vi "GenerateSelectorBounds.vi"(8 "error in (no error)":errorcluster, 10 "Master Bounds Rect":T1, 11 "MultiFrameStructure in":refnum<vi>) -> (0 "error out":errorcluster, 2 "JSON string":string, 3 "reference out":refnum<vi>)   [LabVIEW 2017]
uses:
  <vilib>/Utility/miscctls.llb/LVRectTypeDef.ctl
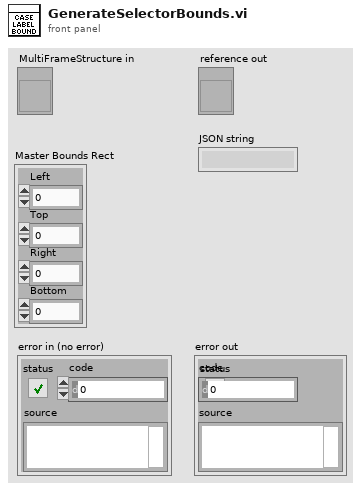
[diagram p1: front panel]
types:
  T1 = typedef "LVRectTypeDef.ctl" = cluster{"Left":i16, "Top":i16, "Right":i16, "Bottom":i16}
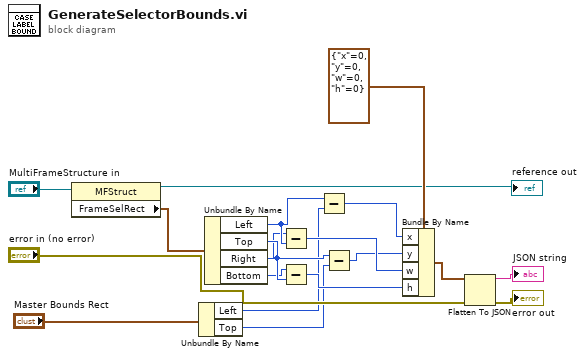
[diagram p0: block diagram]
diagram:
  n1 = property class="MFStruct"(reference="MultiFrameStructure in") -> (reference out=→"reference out":refnum<vi>, "FrameSelRect"=w4:T1)  [unwired: 1 in, 1 out]
  n2 = Unbundle By Name("Master Bounds Rect") -> ("Left"=w7:i16, "Top"=w9:i16)
  n3 = Unbundle By Name(w4) -> ("Left"=w8:i16, "Top"=w10:i16, "Right"=w5:i16, "Bottom"=w6:i16)
  n4 = Subtract(x=w5, y=w8) -> (x-y=w14:i16)
  n5 = Subtract(x=w6, y=w10) -> (x-y=w15:i16)
  n6 = Subtract(x=w8, y=w7) -> (x-y=w12:i16)
  n7 = Subtract(x=w10, y=w9) -> (x-y=w13:i16)
  n8 = Bundle By Name(cluster=cluster{"x":i32, "y":i32, "w":i32, "h":i32} {"x"=0, "y"=0, "w"=0, "h"=0}, "x"=w12, "y"=w13, "w"=w14, "h"=w15) -> (w16:cluster{"x":i32, "y":i32, "w":i32, "h":i32})
  n9 = Flatten To JSON(anything=w16, error in (no error)="error in (no error)") -> (JSON string=→"JSON string":string, 11:→"error out":errorcluster)  [unwired: 1 in]
